vi "Set SA Path.vi"(0 "SA 8GHz Path in":refnum<class "SA 8GHz Path.lvclass">, 11 "error in":errorcluster) -> (4 "SA 8GHz Path out":refnum<class "SA 8GHz Path.lvclass">, 15 "error out":errorcluster)   [LabVIEW 2023, in "RFFixtureCharact.RMM.lvlib" / "SA 8GHz Path.lvclass"]
uses:
  Public/Base Classes/Scalar/SA Abstract Path/SA Abstract Path.lvclass/SA Abstract Path.ctl
  Public/Base Classes/Scalar/SA Abstract Path/Properties/Read RFmx Session.vi
  SA 8GHz Path.lvclass
  SA 8GHz Path.lvclass/SA 8GHz Path.ctl
  <resource>/objmgr/RFmxSpecAn.rc
  Public/Base Classes/Scalar/SA Path/SA Path.lvclass
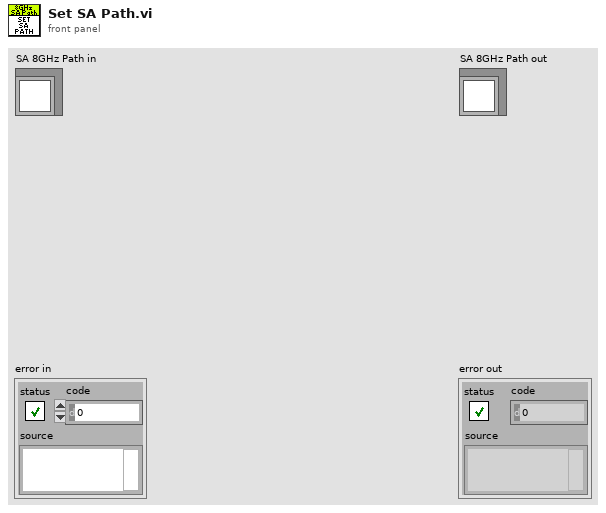
[diagram p1: front panel]
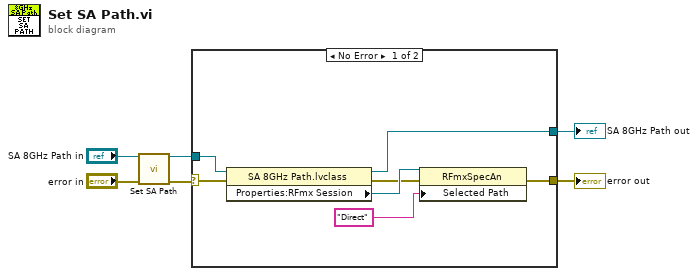
[diagram p0: block diagram]
diagram:
  n1 = call-parent "Set SA Path.vi"("SA Path in"="SA 8GHz Path in", "error in"="error in") -> ("SA Path out"=w1:refnum<class "SA 8GHz Path.lvclass">, "error out"=w2:errorcluster)  [unwired: 12 in]
  n2 = case shown="No Error" w2 {
    selector: w2 -> [w13 w15]
    tunnel: w1 -> [w12 w14]
    tunnel: [w11 w14] -> w4
    tunnel: [w8 w15] -> w3
    frame No Error {
      n3 = property class="SA 8GHz Path.lvclass"(reference=w12, error in=w13) -> (reference out=w11:refnum<class "SA 8GHz Path.lvclass">, error out=w9:errorcluster, "Properties:RFmx Session"=w10:refnum<k21>)
      n4 = property class="RFmxSpecAn"(reference=w10, error in=w9, "Selected Path"="Direct") -> (error out=w8:errorcluster)  [unwired: 1 out]
    }
    frame Error {
    }
  }
  "error out" <- w3
  "SA 8GHz Path out" <- w4
